vi "IMP.vi"(0 "System no.":i32=1 min=1 max=4 step=1, 2 "Axis to command":string, 3 "Impulse size":dbl caption="Numeric" format="%.6f", 4 "No.of digits":i16=4, 5 "error in":errorcluster) -> (19 "error out":errorcluster)   [LabVIEW 2020]
doc: "Performs a single impulse-move (two equal moves in opposite directions in quick succession) from the current position with specified impulse size (amplitude) and records a fixed number of actual positions at specified intervals thereafter, which can be read out with IMP?.vi (GCS 1.0) or DRR?.vi (GCS 2.0). If supported, \"Delay\" sets the number of servo loops between each position recording. \n\nE-517, E-518: Controller saves up to 8,192 position values. Typically, IMP is used in open-loop mode. For a single step-move, see STE.vi . Use DRR?.vi to read recorded values back. The number of servo cycles used for data recording depends on the setting made with RTR.Motion commands like IMP are not allowed when the controller is in OFFLINE mode or when the wave generator output is active. When a macro is running on the controller, IMP will be executed not until the macro is finished or stopped. See \"Control Value Generation\" and \"Control Modes\" in the controller User manual for details.\n\nC-413, E-709: Controller saves up to 4096 position values. Typically, IMP is used in open-loop mode. For a single step-move, see \"STE.vi\". Use DRR?.vi to read recorded values back. The number of servo cycles used for data recording depends on the setting made with RTR. Motion commands are not allowed when the wave generator is active or the analog input is used for target generation.\n\nE-710: Delay = 0. Controller saves 32,256 position values. Width of impulse and sampling interval taken from \"Table rate\" parameter, set with SPA_Hex.vi. Caution: \"Table rate\" parameter influences wave generator also, not only IMP. For a single step-move, see STE.vi. Use IMP?.vi to read position values back.\n\nE-712: Delay = 0. Controller saves up to 262,144 position values. Typically, IMP is used in open-loop mode. For a single step-move, see STE.vi. Use DRR?.vi to read recorded values back. The number of servo cycles used for data recording depends on the setting made with RTR. Motion commands are not allowed when a wave generator is active or the analog input is used for target generation.\n\nE-725, E-727: Delay = 0. Controller saves up to 262,144 position values. Typically, IMP is used in open-loop mode. For a single step-move, see STE.vi. Use DRR?.vi to read recorded values back. The number of servo cycles used for data recording depends on the setting made with RTR. Motion commands are not allowed when a wave generator is active or the analog input is used for target generation.\n\nE-753: Controller saves up to 65,536 position values. Typically, IMP is used in open-loop mode. For a single step-move, see STE.vi. Use DRR?.vi to read recorded values back. The number of servo cycles used for data recording depends on the setting made with RTR. Motion commands are not allowed when the wave generator is active or the analog input is used for target generation.\n\nE-754: Delay = 0. Controller saves up to 1,048,576 position values. Typically, IMP is used in open-loop mode. For a single step-move, see STE.vi. Use DRR?.vi to read recorded values back. The number of servo cycles used for data recording depends on the setting made with RTR. Motion commands are not allowed when a wave generator is active or the analog input is used for target generation.\n\nE-755: Delay= 0. Controller saves 4,096 position values. Typically, IMP is used in open-loop mode. For a single step-move, see STE.vi. Use DRR?.vi to read recorded values back.\n\nE-761: Delay is impuls width in servo loops. Default value is 0 (for one servo loop). Controller saves 8,192 position values. Typically, IMP is used in open loop mode. For a single step-move, see STE.vi. The number of servo cycles used for data recording depends on the setting made with RTR.vi. Use DRR?.vi or IMP?.vi to read position values back.\n\nC-887, F-206, M-8X0: Only for GCS syntax version = GCS 2.0 or higher (Check with CSV?.vi. If CSV?.vi is not supported, syntax version is GCS 1.0). See controller user manual for number of points (can be changed by setting the appropriate parameter value). For a single step-move, see STE.vi. Use DRR?.vi to read recorded values back."
uses:
  Communication/Global1.vi
panel:
  in  "Delay":i32 caption="Numeric"
  # "Performs a single impulse-move (two equal moves in opposite\ndirections in quick succession) from the current position with\nspecified impulse size (amplitude) and records a fixed number \nof actual positions at specified intervals thereafter, which can \nbe read out with IMP?.vi (GCS 1.0) or DRR?.vi (GCS 2.0). \"Delay\"\nsets the number of servo loops between each position recording."
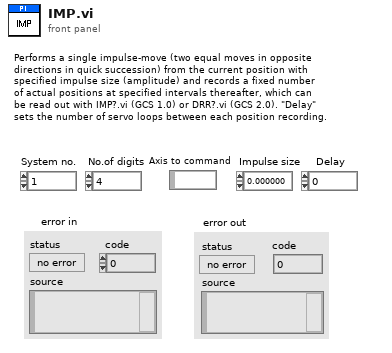
[diagram p1: front panel]
types:
  T1 = typedef "Syntax.ctl" = enum16{"GCS 1.0", "GCS 2.0", "GCS 3.0"}
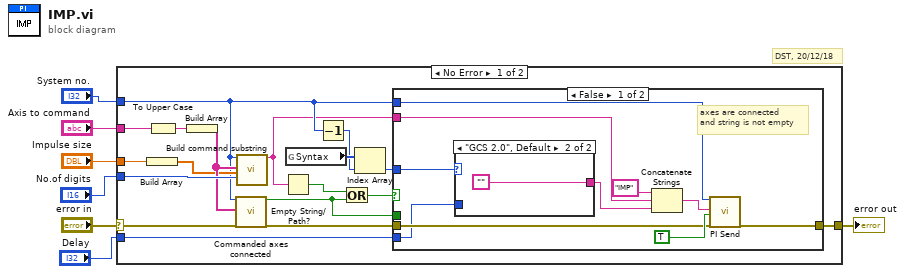
[diagram p0: block diagram]
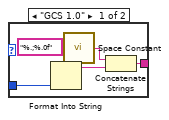
[diagram p2: hidden frame]
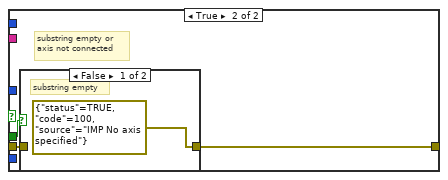
[diagram p3: hidden frame]
diagram:
  # "DST, 20/12/18"
  n1 = case shown="No Error" "error in" {
    selector: "error in" -> [w12 w47]
    tunnel: [w25 w47] -> w7
    tunnel: "No.of digits" -> [w24 _]
    tunnel: "System no." -> [w13 _]
    tunnel: "Impulse size" -> [w20 _]
    tunnel: "Axis to command" -> [w18 _]
    tunnel: "Delay" -> [w16 _]
    frame No Error {
      n2 = Build Array(w20) -> (w19:dbl[])
      n3 = To Upper Case(1:w18) -> (0:w17:string)
      n4 = Build Array(w17) -> (w21:string[])
      n5 = call "Commanded axes connected.vi"("System no."=w13, "Commanded axes"=w21, "error in"=w12) -> ("Controller error"=w9:bool, "error out"=w23:errorcluster)  [unwired: 1 in, 14 out]
      n6 = call "Build command substring.vi"("System no."=w13, "Affected axes"=w21, "Parameters"=w19, "No. of digits"=w24) -> ("Command substring"=w11:string)  [unwired: 3 in, 12 out]
      n7 = Empty String/Path?(string/path=w11) -> (empty?=w10:bool)
      n8 = global read "Global1.vi" "Syntax"() -> (w15:T1[])
      n9 = Decrement(x=w13) -> (x-1=w14:i32)
      n10 = Or(x=w10, y=w9) -> (x .or. y?=w22:bool)
      n11 = Index Array(array=w15, index=w14) -> (element=w8:T1)
      n12 = case shown="False" w22 {
        tunnel: w11 -> [w34 _]
        tunnel: [w30 w44] -> w25
        tunnel: w23 -> [w31 w42]
        tunnel: w9 -> [_ w43]
        tunnel: w13 -> [w29 _]
        tunnel: w16 -> [w28 _]
        tunnel: w8 -> [w26 _]
        frame False {
          # "axes are connected \nand string is not empty"
          n13 = case shown="\"GCS 2.0\", Default" w26 {
            tunnel: w28 -> [w39 _]
            tunnel: [w36 ""] -> w27
            frame "GCS 1.0" {
              n14 = Format Into String(format string="%.;%.0f" ("Format String"), w39) -> (resulting string=w37:string)  [unwired: 2 in, 1 out]
              n15 = call <vilib>:"Space Constant.vi"() -> ("String"=w38:string)
              n16 = Concatenate Strings(w38, w37) -> (w36:string)
            }
            frame "GCS 2.0", Default {
            }
          }
          n17 = Concatenate Strings("IMP", w34, w27) -> (w32:string)
          n18 = call "PI Send.vi"("System no."=w29, "String to send"=w32, "Attach termination char.?"=TRUE ("Attach Linefeed?"), "error in"=w31) -> ("error out"=w30:errorcluster)  [unwired: 2 in, 13 out]
        }
        frame True {
          # "substring empty or \naxis not connected"
          n19 = case shown="False" w43 {
            tunnel: [errorcluster {"status"=TRUE, "code"=100, "source"="IMP No axis specified"} ("error out") w46] -> w44
            tunnel: w42 -> [_ w46]
            frame False {
              # "substring empty"
            }
            frame True {
              # "commanded axis not connected"
            }
          }
        }
      }
    }
    frame Error {
    }
  }
  "error out" <- w7
